vi "watchPress_01.vi"() -> ()   [LabVIEW 2011]
panel:
  in  "interval (s)":dbl=1.0
  in  "stop":bool
  out "P(Torr)":string
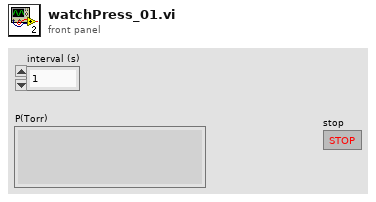
[diagram p1: front panel]
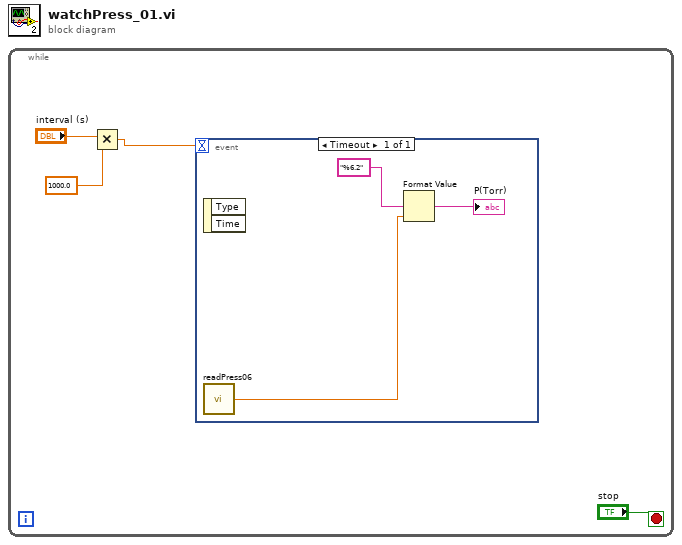
[diagram p0: block diagram]
diagram:
  n1 = while {
    stop <- "stop" stop-if-true
    n2 = Multiply(x="interval (s)", y=1000.0) -> (x*y=w2:dbl)
    n3 = event shown="[0] Timeout" {
      selector: _ -> [_]
      dyn-events: _ -> [_]
      timeout: w2 -> [_]
      event Timeout {
        n4 = event-data() -> ()  [unwired: 1 in, 2 out]
        n5 = call "readPress06.vi"() -> ("P"=w6:dbl)
        n6 = Format Value(format string="%6.2", value (0)=w6) -> (output string=→"P(Torr)":string)  [unwired: 1 in]
      }
    }
  }
